vi "report_module.vi"(8 "error in (no error)":errorcluster, 9 "manual_save":bool, 10 "report_data":string[](array[string]), 11 "Instrument in":refnum<class "Instrument.lvclass">) -> (0 "error out":errorcluster, 3 "Instrument out":refnum<class "Instrument.lvclass">)   [LabVIEW 2019, in "Instrument.lvclass"]
uses:
  Instrument.lvclass
  Instrument.lvclass/Instrument.ctl
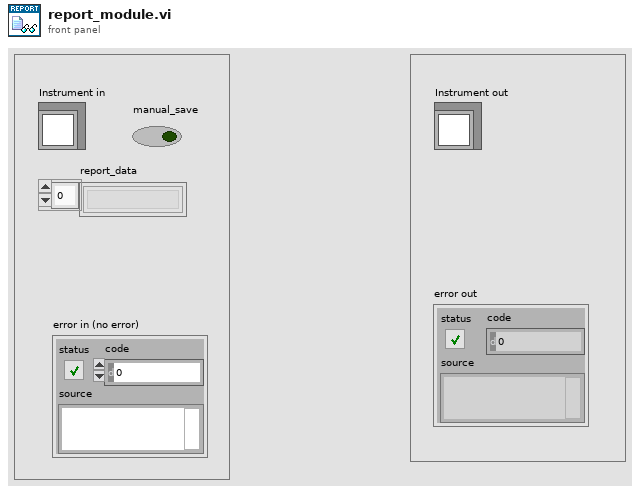
[diagram p1: front panel]
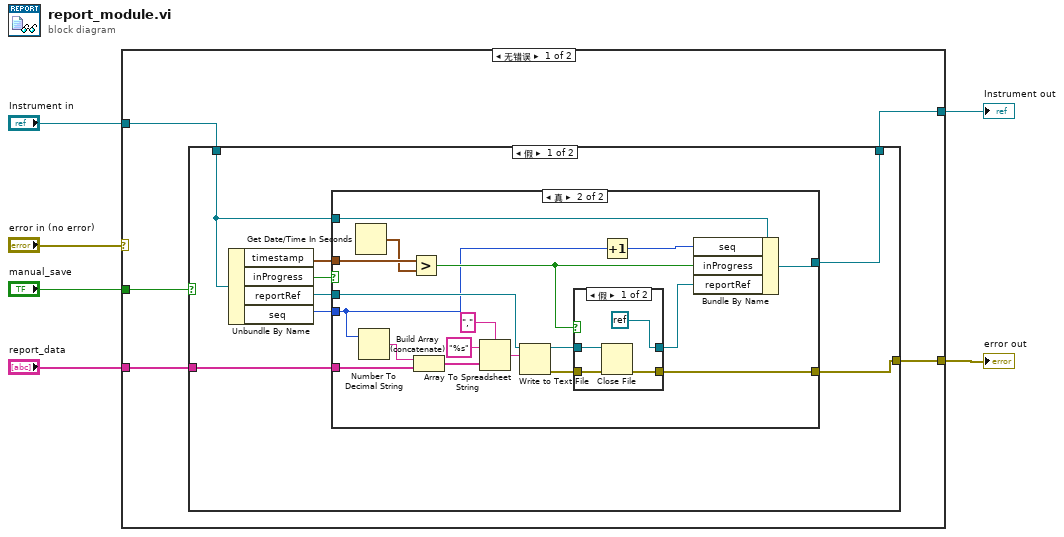
[diagram p0: block diagram]
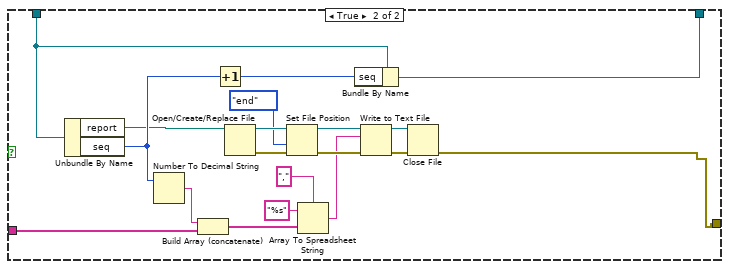
[diagram p4: hidden frame]
diagram:
  n1 = case shown="无错误" "error in (no error)" {
    selector: "error in (no error)" -> [_ w64]
    tunnel: "report_data" -> [w11 _]
    tunnel: [w10 w64] -> w5
    tunnel: "manual_save" -> [w9 _]
    tunnel: "Instrument in" -> [w8 w65]
    tunnel: [w7 w65] -> w2
    frame No Error {
      n2 = case shown="假" w9 {
        tunnel: w11 -> [w15 w47]
        tunnel: w8 -> [w14 w53]
        tunnel: [w12 w45] -> w10
        tunnel: [w17 w52] -> w7
        frame False {
          n3 = Unbundle By Name(w14) -> ("timestamp"=w19:timestamp, "inProgress"=w18:bool, "reportRef"=w16:refnum<file>, "seq"=w13:i32)
          n4 = case shown="真" w18 {
            tunnel: w19 -> [_ w38]
            tunnel: [w20 w28] -> w17
            tunnel: w16 -> [_ w36]
            tunnel: w15 -> [_ w21]
            tunnel: [_ w30] -> w12
            tunnel: w14 -> [w20 w29]
            tunnel: w13 -> [_ w24]
            frame False {
            }
            frame True {
              n5 = Get Date/Time In Seconds() -> (seconds since 1Jan1904=w37:timestamp)
              n6 = Number To Decimal String(number=w24) -> (decimal integer string=w22:string)  [unwired: 1 in]
              n7 = Greater?(x=w38, y=w37) -> (0:w27:bool)
              n8 = Build Array (concatenate)(w22, w21) -> (w23:string[])
              n9 = Array To Spreadsheet String(delimiter (Tab)=",", array=w23, 3:"%s" ("format string")) -> (spreadsheet string=w32:string)
              n10 = Write to Text File(file (use dialog)=w36, text=w32) -> (refnum out=w31:refnum<file>, error out=w35:errorcluster)  [unwired: 2 in, 1 out]
              n11 = case shown="假" w27 {
                tunnel: w35 -> [w42 w43]
                tunnel: w31 -> [w41 w44]
                tunnel: [w40 w43] -> w30
                tunnel: [refnum<k0> refnum w44] -> w26
                frame False {
                  n12 = Close File(refnum=w41, error in=w42) -> (error out=w40:errorcluster)  [unwired: 1 out]
                }
                frame True {
                }
              }
              n13 = Increment(x=w24) -> (x+1=w25:i32)
              n14 = Bundle By Name(cluster=w29, "seq"=w25, "inProgress"=w27, "reportRef"=w26) -> (w28:refnum<class "Instrument.lvclass">)
            }
          }
        }
        frame True {
          n15 = Unbundle By Name(w53) -> ("report"=w49:path, "seq"=w51:i32)
          n16 = Number To Decimal String(number=w51) -> (decimal integer string=w54:string)  [unwired: 1 in]
          n17 = Build Array (concatenate)(w54, w47) -> (w48:string[])
          n18 = Increment(x=w51) -> (x+1=w50:i32)
          n19 = Open/Create/Replace File(file path (use dialog)=w49) -> (refnum out=w61:refnum<file>, error out=w58:errorcluster)  [unwired: 5 in, 1 out]
          n20 = Set File Position(refnum=w61, from (0:start)=enum16{"start", "end", "current"}."end", error in=w58) -> (refnum out=w60:refnum<file>, error out=w57:errorcluster)  [unwired: 1 in]
          n21 = Array To Spreadsheet String(delimiter (Tab)=",", array=w48, 3:"%s" ("format string")) -> (spreadsheet string=w46:string)
          n22 = Bundle By Name(cluster=w53, "seq"=w50) -> (w52:refnum<class "Instrument.lvclass">)
          n23 = Write to Text File(file (use dialog)=w60, text=w46, error in=w57) -> (refnum out=w56:refnum<file>, error out=w55:errorcluster)  [unwired: 1 in, 1 out]
          n24 = Close File(refnum=w56, error in=w55) -> (error out=w45:errorcluster)  [unwired: 1 out]
        }
      }
    }
    frame Error {
    }
  }
  "error out" <- w5
  "Instrument out" <- w2
